vi "PID_3Tanks.vi"() -> ()   [LabVIEW 2014]
uses:
  <vilib>/Simulation/Scripting/Companion Diagram/SimConfigNode/SimParams.ctl
  <vilib>/Simulation/Scripting/Companion Diagram/SimConfigNode/_simSolvers.ctl
  <vilib>/Simulation/Implementation/Shared/SIMSCR Execution Mode.ctl
  <vilib>/Simulation/Param Hierarchy/Typedefs/SIMPH Param Control Actions.ctl
  <vilib>/Simulation/Implementation/Shared/SIM limit type.ctl
  <vilib>/Simulation/Implementation/Shared/NILVSim_ParamChanged.vi
  <vilib>/Simulation/Implementation/Shared/NILVSIM_BeginStep.vi
  <vilib>/Simulation/DataSources/Implementation/NILVSim Step.llb/SIM Step (scalar).vi
  <vilib>/Simulation/ContinuousLinear/Implementation/NILVSim Transport Delay.llb/SIM Transport Delay Distributor (scalar).vi
  <vilib>/Simulation/ContinuousLinear/Implementation/NILVSim Integrator new.llb/SIM Integrator distributor (scalar).vi
  <vilib>/Simulation/ContinuousLinear/Implementation/NILVSim Integrator new.llb/SIM Integrator collector (scalar).vi
  <vilib>/Simulation/ContinuousLinear/Implementation/NILVSim Derivative.llb/SIM derivative (scalar).vi
  <vilib>/Simulation/ContinuousLinear/Implementation/NILVSim Transport Delay.llb/SIM Transport Delay Collector (scalar).vi
  <vilib>/Simulation/SignalDisplay/Implementation/NILVSim Time Waveform.llb/SIM Time Waveform (vector).vi
  <vilib>/Simulation/Implementation/Shared/NILVSim_Manager.vi
  <vilib>/Utility/error.llb/Clear Errors.vi
  <vilib>/Simulation/Implementation/Shared/NILVSim_FinalizeModel.vi
  <vilib>/Simulation/Implementation/Shared/SIM Unbundle Sim Info.vi
  <vilib>/Simulation/Implementation/Shared/NILVSim_Initialize.vi
  <vilib>/imath/engines/lvmath2/RunTimeEngine/NodeEndStatement/NIMS_NodeEndStatement_Output.vi
  <instcachedir>/0/NIMS_NodeEndStatement_Output_53EC0D466D134D7ABD903AC30B43404B.lvgen/NIMS_NodeEndStatement_Output_53EC0D466D134D7ABD903AC30B43404B_001.vi
  <vilib>/imath/engines/lvmath2/RunTimeEngine/ErrorHandling/NIMS_Finalize Error.vi
  <vilib>/Simulation/Utility/Implementation/NILVSim Get Time and IsAcceptedStep.vi
  <vilib>/Simulation/Implementation/Shared/SIMSH Read Queue.vi
  <vilib>/Simulation/Implementation/Shared/NILVSim_GetModelError.vi
  <vilib>/Simulation/Implementation/Shared/SIM Bundle Sim Info.vi
  <vilib>/Simulation/Scripting/Companion Diagram/SimConfigNode/SimDog.xnode
  <vilib>/Simulation/Implementation/XNodeFramework/SimXNode/SimX.xnode
  <vilib>/Simulation/ContinuousLinear/Implementation/NILVSim Integrator new.llb/SIM Integrator (scalar).vi
  <vilib>/Simulation/ContinuousLinear/Implementation/NILVSim Transport Delay.llb/SIM Transport Delay Indirect (scalar).vi
  <vilib>/Simulation/Implementation/Shared/NI_SIM_Implementation.lvlib
panel:
  out "Valvula-3":dbl=1.2247448713915863
  out "ISE 3":dbl=0.9791589484430331
  in  "factor Kc3":dbl=0.65
  in  "factor Td3":dbl=0.75
  out "Tank Control ZN CL":dbl(slide)=1.4999999999999512 scale=0.0..2.0
  in  "factor Ti3":dbl=1.15
  out "Td3":dbl=1.0
  out "Ti3":dbl=4.0
  out "Kc3":dbl=0.69
  in  "Tu3":dbl=8.0
  in  "Ku3":dbl=1.15
  in  "Flujo inicial en tuberia":dbl=1.0
  in  "H0":dbl=1.0
  in  "Href":dbl=1.5
  out "Valvula-2":dbl=1.2247448713915958
  out "Perturbacion":dbl caption="ISE 2"
  in  "factor Ti2":dbl=1.0
  out "Tank  Control AMIGO":dbl(slide)=1.4999999999999867 scale=0.0..2.0
  in  "factor Td2":dbl=1.0
  in  "factor Kc2":dbl=1.2
  out "ISE 2":dbl=1.0875092978295866
  out "ISE 1":dbl=0.9692441486635541
  out "Valvulas":waveform(dbl)[](graph)=[{"t0"=timestamp(150 s since 1904-01-01), "dt"=1.0, "Y"=[1.2247448713915836]}, {"t0"=timestamp(150 s since 1904-01-01), "dt"=1.0, "Y"=[1.2247448713915958]}, {"t0"=timestamp(150 s since 1904-01-01), "dt"=1.0, "Y"=[1.224744871391586]}]
  in  "factor Kc1":dbl=1.2
  in  "factor Td1":dbl=0.75
  in  "Amplitud perturbacion":dbl
  out "Td2":dbl=1.0344827586206897
  out "Ti2":dbl=2.625
  out "Kc2":dbl=0.23809523809523808
  out "Td1":dbl=1.5
  out "Ti1":dbl=6.0
  out "Kc1":dbl=0.38095238095238093
  in  "tp":dbl=2.0
  in  "Tt":dbl=3.0
  in  "Kp":dbl=2.1
  out "ISE":waveform(dbl)[](graph)=[{"t0"=timestamp(150 s since 1904-01-01), "dt"=1.0, "Y"=[0.9692441486635541]}, {"t0"=timestamp(150 s since 1904-01-01), "dt"=1.0, "Y"=[1.0875092978295866]}, {"t0"=timestamp(150 s since 1904-01-01), "dt"=1.0, "Y"=[0.9791589484430331]}]
  out "Tank Control ZN O.L.":dbl(slide)=1.5000000000000084 scale=0.0..2.0
  in  "K1":dbl=1.0
  in  "A1":dbl=1.0
  in  "factor Ti1":dbl=0.75
  out "Alturas":waveform(dbl)[](graph)=[{"t0"=timestamp(150 s since 1904-01-01), "dt"=1.0, "Y"=[1.5000000000000084]}, {"t0"=timestamp(150 s since 1904-01-01), "dt"=1.0, "Y"=[1.4999999999999867]}, {"t0"=timestamp(150 s since 1904-01-01), "dt"=1.0, "Y"=[1.4999999999999512]}]
  # "Diseño de controladores de altura de un depósito"
  # "Altura de Referencia"
  # "PERTURBACIÓN"
  # "CONTROLADORES PID"
  # "SISTEMA"
  # "IDENTIFICACIÓN"
  # "Ziegler-Nichols O.L."
  # "AMIGO"
  # "Ziegler-Nichols C.L."
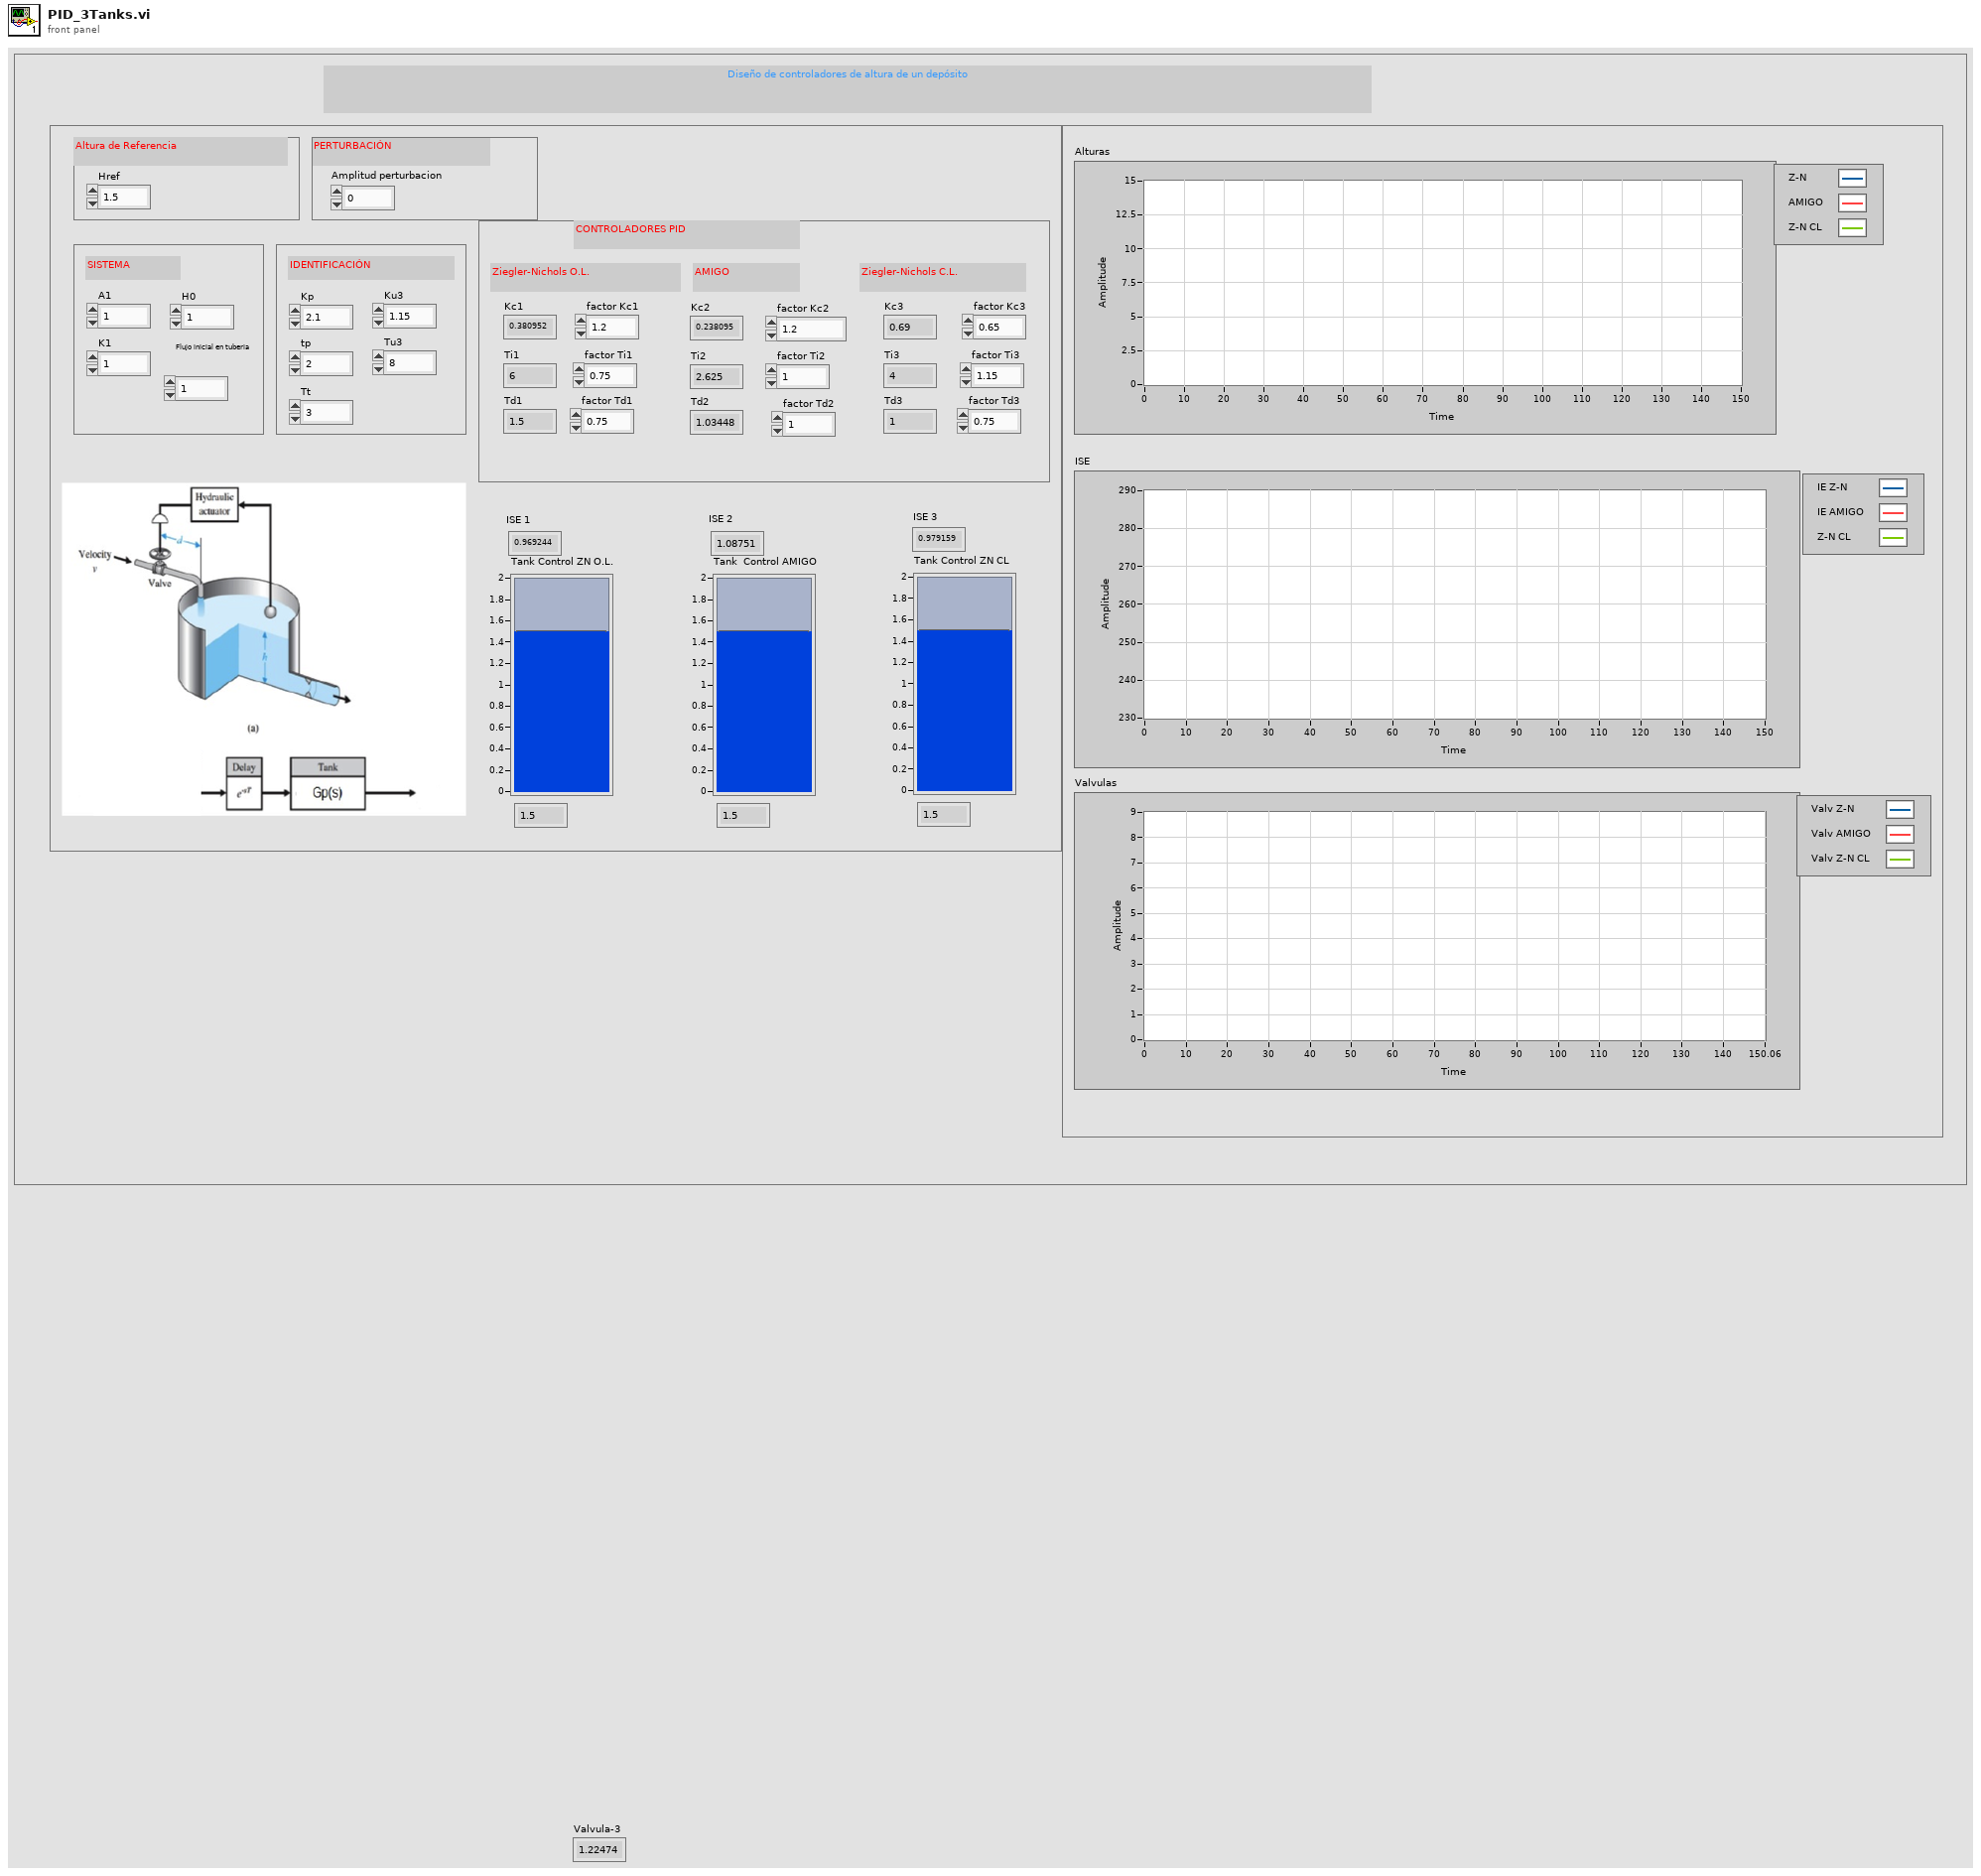
[diagram p1: front panel]
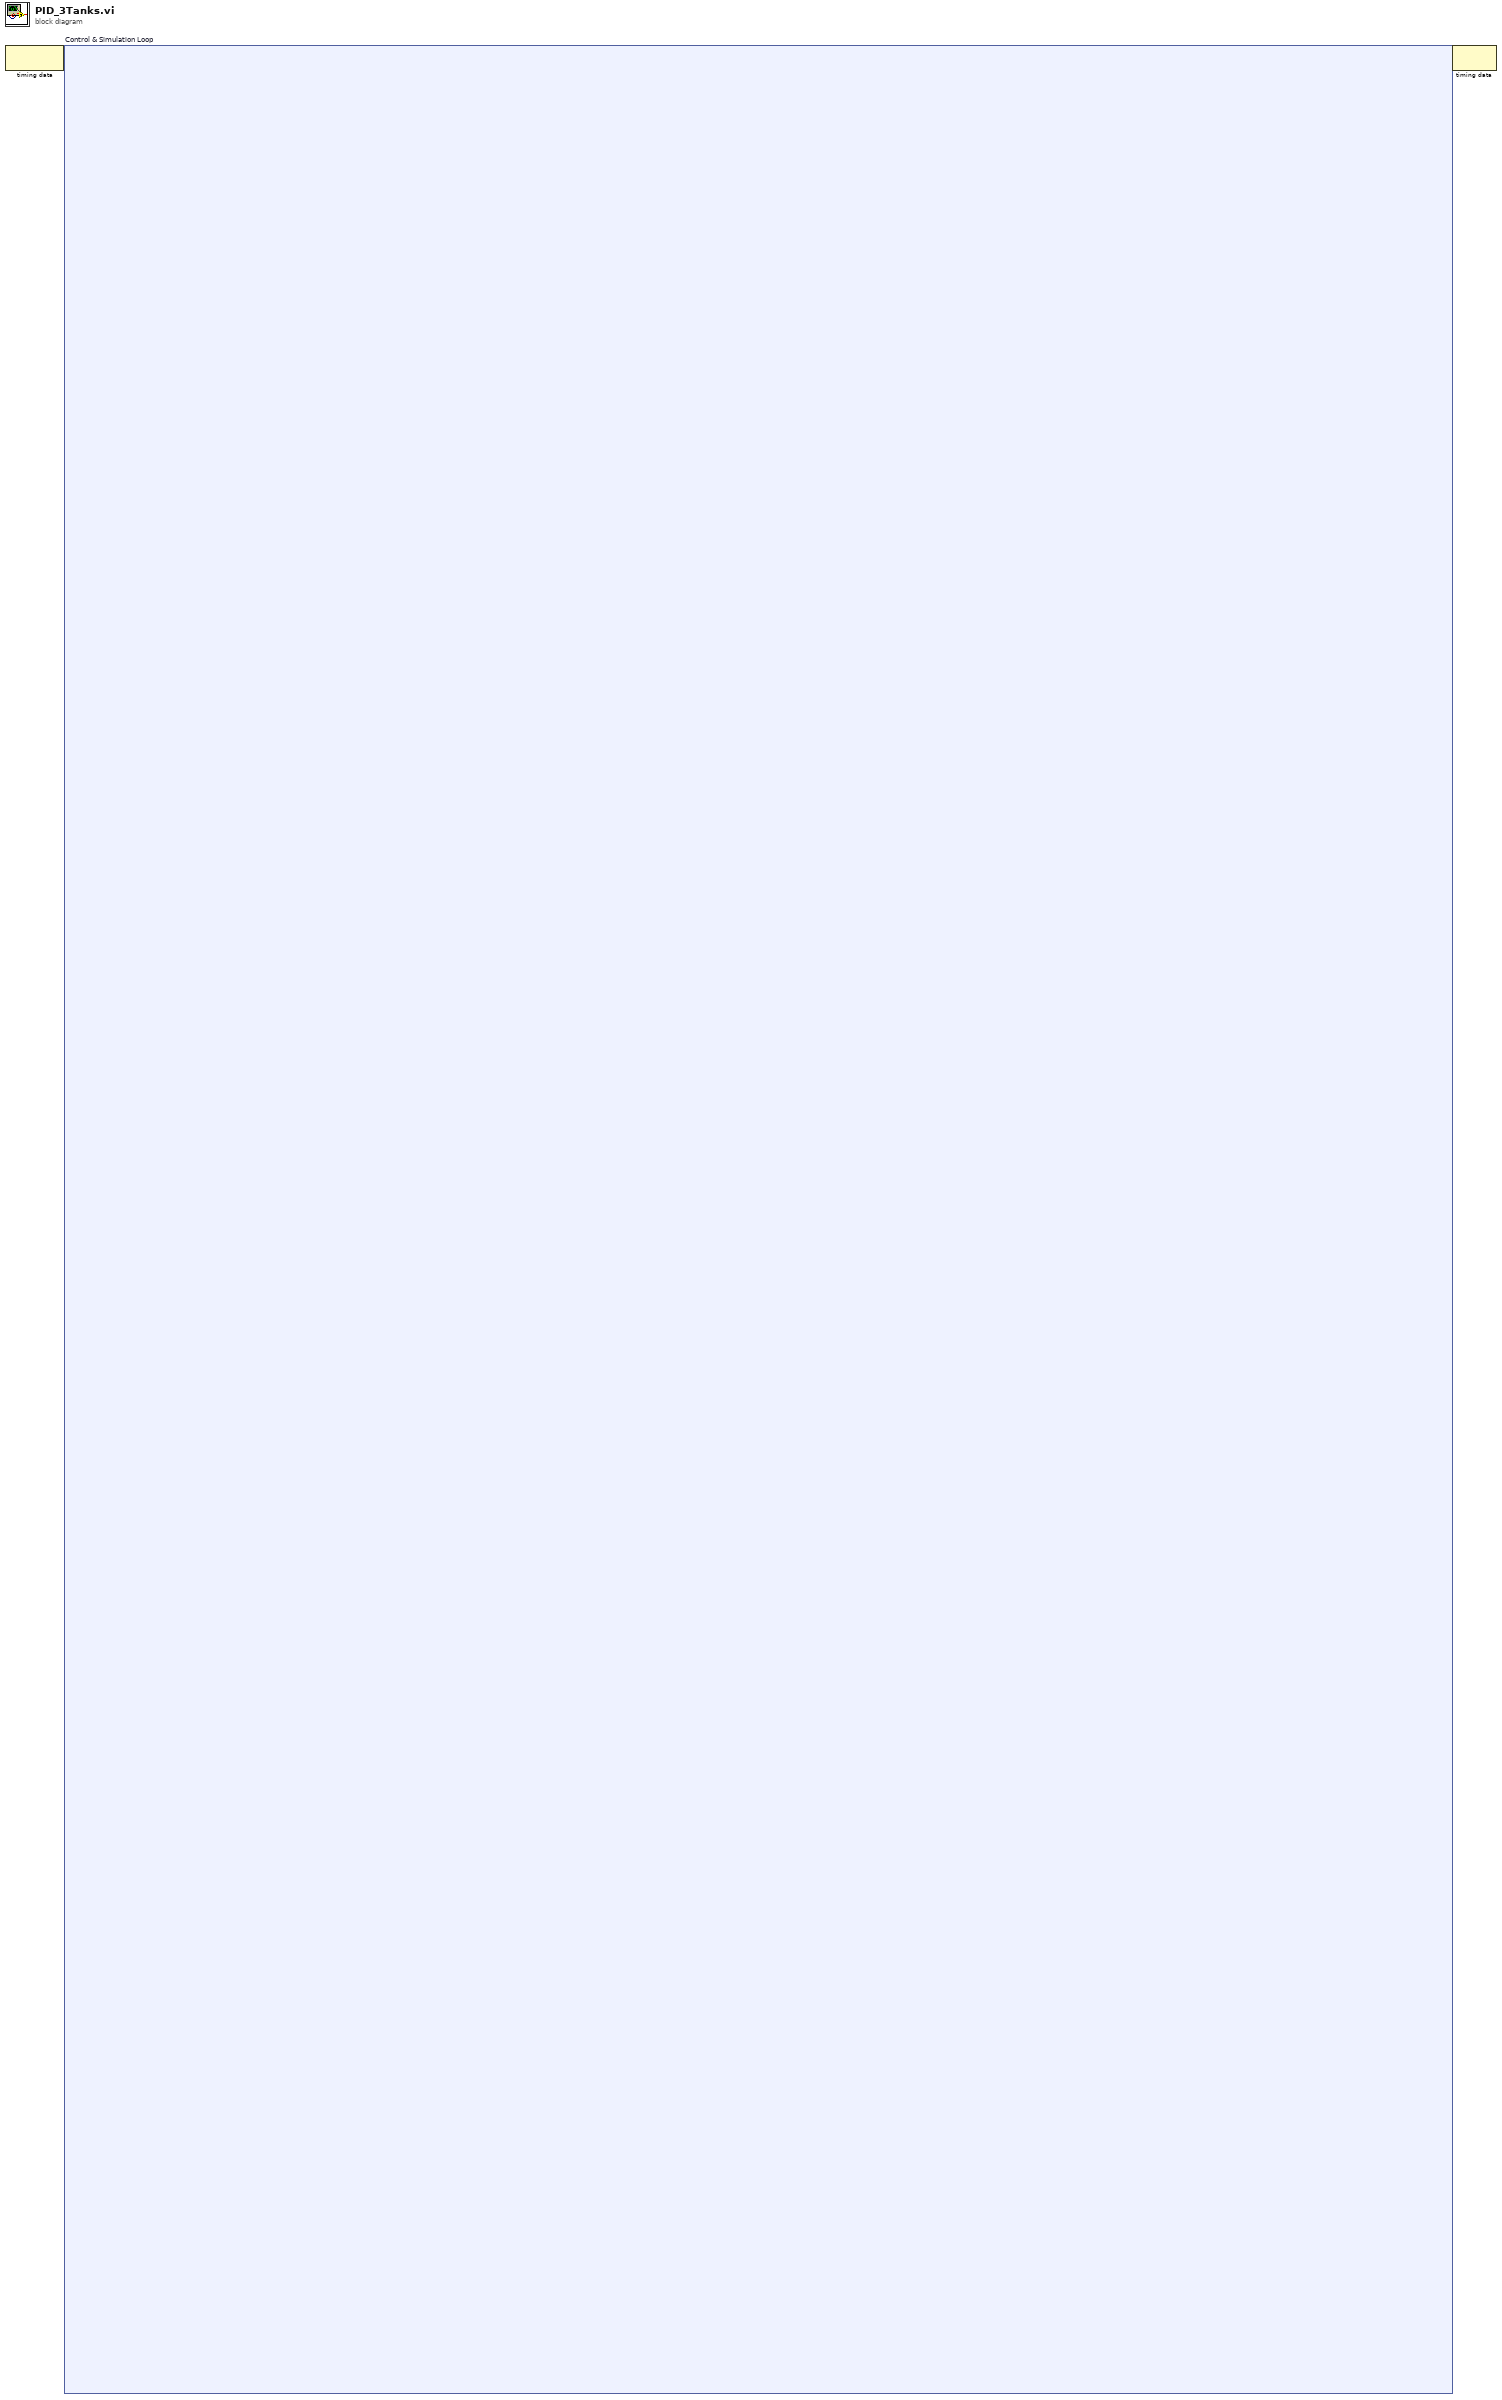
[diagram p0: block diagram]
diagram:
  n1 = node-c288() -> (w2:variant)  [unwired: 1 in]
  n2 = node-c254 "Control & Simulation Loop"(w2) -> (w1:variant)
  n3 = node-c288(w1) -> ()  [unwired: 1 out]
